vi "communications_configuration.vi"(4 "Comms":string(combo)="330", 5 "Protocol":string(combo)="0", 6 "Separation char (Omega protocol, continuous data mode)":string(combo)="0", 7 "Data mode":string(combo)="0", 8 "error in (no error)":errorcluster, 9 "Response echo enabled":string(combo)="0", 10 "Line feed enabled":string(combo)="0", 11 "VISA Refnum in":refnum<visa-resource-name>) -> (0 "error out":errorcluster, 3 "VISA Refnum out":refnum<visa-resource-name>)   [LabVIEW 2018]
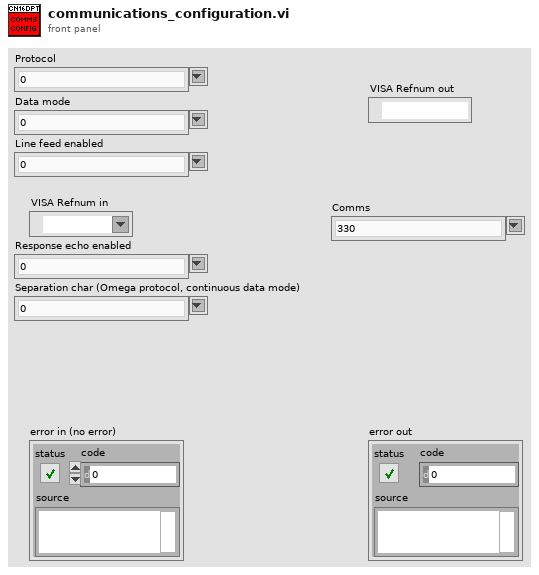
[diagram p1: front panel]
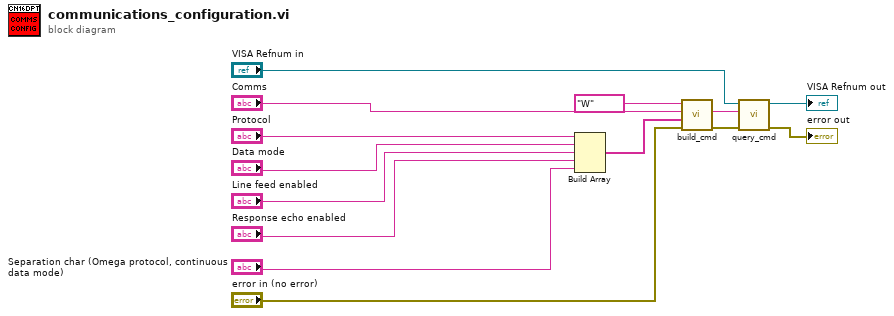
[diagram p0: block diagram]
diagram:
  n1 = Build Array("Protocol", "Data mode", "Line feed enabled", "Response echo enabled", "Separation char (Omega protocol, continuous data mode)") -> (w10:string[])
  n2 = call "build_cmd.vi"("error in (no error)"="error in (no error)", "Parameter list"=w10, "Command ID"="Comms", "Command class"="W") -> ("error out"=w8:errorcluster, "Command"=w7:string)  [unwired: 6 in]
  n3 = call "query_cmd.vi"("error in (no error)"=w8, "Command"=w7, "VISA resource name"="VISA Refnum in") -> ("error out"=→"error out":errorcluster, "VISA resource name out"=→"VISA Refnum out":refnum<visa-resource-name>)  [unwired: 6 in, 1 out]
